vi "Periodic Tasks.vi"(8 "error in":errorcluster) -> ()   [LabVIEW 2017]
doc: "This VI runs in parallel to other tasks. It can contain as many user-defined periodic loops as you need. These can carry out PID or other sorts of timed response."
uses:
  <vilib>/Rock Robotics/WPI/DriverStation/WPI_DriverStationRobotMode2.ctl
  <vilib>/Rock Robotics/WPI/Solenoid/WPI_SolenoidValue.ctl
  <vilib>/Rock Robotics/WPI/ThirdParty/Phoenix-LabVIEW/Motor Controller/Controls/CTRE_Phoenix_MotorControl_ControlMode.ctl
  Robot Global Data.vi
  <vilib>/Rock Robotics/WPI/Solenoid/WPI_SolenoidSetEnum.vi
  <vilib>/addons/control/pid/pid.llb/PID (DBL).vi
  <vilib>/Rock Robotics/WPI/Utilities/WPI_GetSetVariantRefNum.vi
  <vilib>/Rock Robotics/WPI/ThirdParty/Phoenix-LabVIEW/Motor Controller/Get/CTRE_Phoenix_MotorController_GetOutputCurrent_Enhanced.vi
  <vilib>/addons/control/pid/NI_PID_pid.lvlib
panel:
  out "Distance":dbl
  out "Distance 2":dbl
  out "Angle":dbl
  out "Normalized Value":dbl
  out "Output Current":dbl
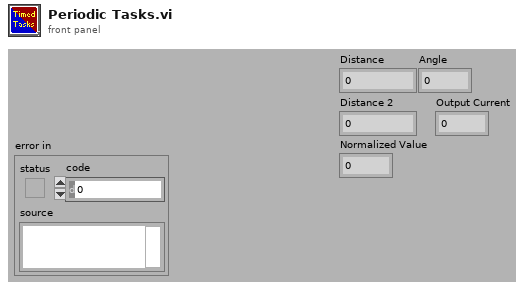
[diagram p1: front panel]
types:
  T1 = typedef "WPI_SolenoidDevRef.ctl" = cluster{"DevStatus":errorcluster, "Pneumatics Control Module":u8, "Forward Solenoid Channel":T2, "Reverse Solenoid Channel":T2}
  T2 = typedef "WPI_SolenoidChannel.ctl" = enum8{"Solenoid 0", "Solenoid 1", "Solenoid 2", "Solenoid 3", "Solenoid 4", "Solenoid 5", "Solenoid 6", "Solenoid 7", "Invalid"}
  T3 = typedef "WPI_MotorControlDeviceRef.ctl" = cluster{"DeviceStatus":errorcluster, "Type":T4, "PWM":cluster{"PWM Channel":T5, "DeadBand":T6}, "CAN":cluster{"Device Number":u8, "SetOutput VI Ref":variant, "GetOutput VI Ref":variant, "Enable VI Ref":variant, "Disable VI Ref":variant, "Data":variant}, "Invert":bool, "DIO PWM":cluster{"PWM \"Enable\" Channel":T5, "DIOChannel":T7, "PWM Rate":dbl}}
  T4 = typedef "WPI_MotorControlType.ctl" = enum16{"PWM", "CAN", "DIO PWM"}
  T5 = typedef "FPGA_DIOPWMChannel.ctl" = enum8{"PWM 0", "PWM 1", "PWM 2", "PWM 3", "PWM 4", "PWM 5", "PWM 6", "PWM 7", "PWM 8", "PWM 9", "PWM MXP 0", "PWM MXP 1", "PWM MXP 2", "PWM MXP 3", "PWM MXP 4", "PWM MXP 5", "PWM MXP 6", "PWM MXP 7", "PWM MXP 8", "PWM MXP 9", "Invalid"}
  T6 = typedef "WPI_PWMDeadband.ctl" = cluster{"Name":string, "maxPositivePwm":i32, "minPositivePwm":i32, "centerPwm":i32, "maxNegativePwm":i32, "minNegativePwm":i32, "angularRange":u16}
  T7 = typedef "FPGA_DIOChannel.ctl" = enum8{"DIO 0", "DIO 1", "DIO 2", "DIO 3", "DIO 4", "DIO 5", "DIO 6", "DIO 7", "DIO 8", "DIO 9", "DIO MXP 0", "DIO MXP 1", "DIO MXP 2", "DIO MXP 3", "DIO MXP 4", "DIO MXP 5", "DIO MXP 6", "DIO MXP 7", "DIO MXP 8", "DIO MXP 9", "DIO MXP 10", "DIO MXP 11", "DIO MXP 12", "DIO MXP 13", "DIO MXP 14", "DIO MXP 15", "SPI Port CS1", "SPI Port CS2", "SPI Port CS3", "SPI Port MISO", "SPI Port MOSI", "Invalid"}
  T8 = typedef "WPI_EncoderDevRef.ctl" = cluster{"DevStatus":errorcluster, "EncoderIndex":T9, "CounterIndex":T10, "DistancePerCount":dbl, "Decoding Type":T11}
  T9 = typedef "FPGA_EncoderIdx.ctl" = enum8{"Enc 0", "Enc 1", "Enc 2", "Enc 3", "Enc 4", "Enc 5", "Enc 6", "Enc 7", "Invalid"}
  T10 = typedef "FPGA_CounterCtrSystemIndex.ctl" = enum8{"Ctr 0", "Ctr 1", "Ctr 2", "Ctr 3", "Ctr 4", "Ctr 5", "Ctr 6", "Ctr 7", "Invalid"}
  T11 = typedef "WPI_EncoderType.ctl" = enum16{"1x", "2x", "4x"}
  T12 = typedef "WPI_JoystickDevRef.ctl" = cluster{"Device":T13}
  T13 = typedef "WPI_JoystickDeviceEnum.ctl" = enum16{"USB 0", "USB 1", "USB 2", "USB 3", "USB 4", "USB 5"}
  T14 = typedef "WPI_SolenoidValue.ctl" = enum16{"Off", "On", "Forward", "Reverse"}
  T15 = cluster{"Axes[0]":dbl, "Axes[1]":dbl, "Axes[2]":dbl, "Axes[3]":dbl, "Axes[4]":dbl, "Axes[5]":dbl, "Axes[6]":dbl, "Axes[7]":dbl, "Axes[8]":dbl}
  T16 = cluster{"X Center":i32, "X Tolerance":i32, "Y Center":i32, "Y Tolderance":i32}
  T17 = typedef "WPI_DriverStationRobotMode2.ctl" = enum16{"Autonomous Disabled", "Autonomous Enabled", "Teleop Disabled", "Teleop Enabled", "Disconnected", "Finish", "Test Disabled", "Test Enabled", "Emergency Stopped"}
  T18 = typedef "CTRE_Phoenix_MotorControl_ControlMode.ctl" = u16
  T19 = typedef "WPI_PotentiometerDevRef.ctl" = cluster{"DevStatus":errorcluster, "Analog Channel":T20, "Invert Output":bool}
  T20 = typedef "FPGA_AIChannel.ctl" = enum8{"AI 0", "AI 1", "AI 2", "AI 3", "AI MXP 0", "AI MXP 1", "AI MXP 2", "AI MXP 3", "Invalid"}
  T21 = typedef "WPI_GyroDevRef.ctl" = cluster{"DevStatus":errorcluster, "Analog Channel":T20, "Gain (VoltsPerDegree/Second)":dbl, "Gyro Type":enum16{"Analog", "XRS450"}, "Handle":i32, "SPI Bus":T22, "Device Found":bool, "Sample Rate":dbl, "Calibrate On Open":bool, "Offset":dbl}
  T22 = typedef "spi_bus.ctl" = enum16{"SPI On-Board, CS0", "SPI On-Board, CS1", "SPI On-Board, CS2", "SPI On-Board, CS3", "SPI MXP", "Invalid"}
  T23 = cluster{"proportional gain (Kc)":dbl, "integral time (Ti, min)":dbl, "derivative time (Td, min)":dbl}
  T24 = cluster{"Lower Limit":dbl, "Lower Position":dbl, "Switch":dbl, "Scale":dbl, "Upper Limit":dbl}
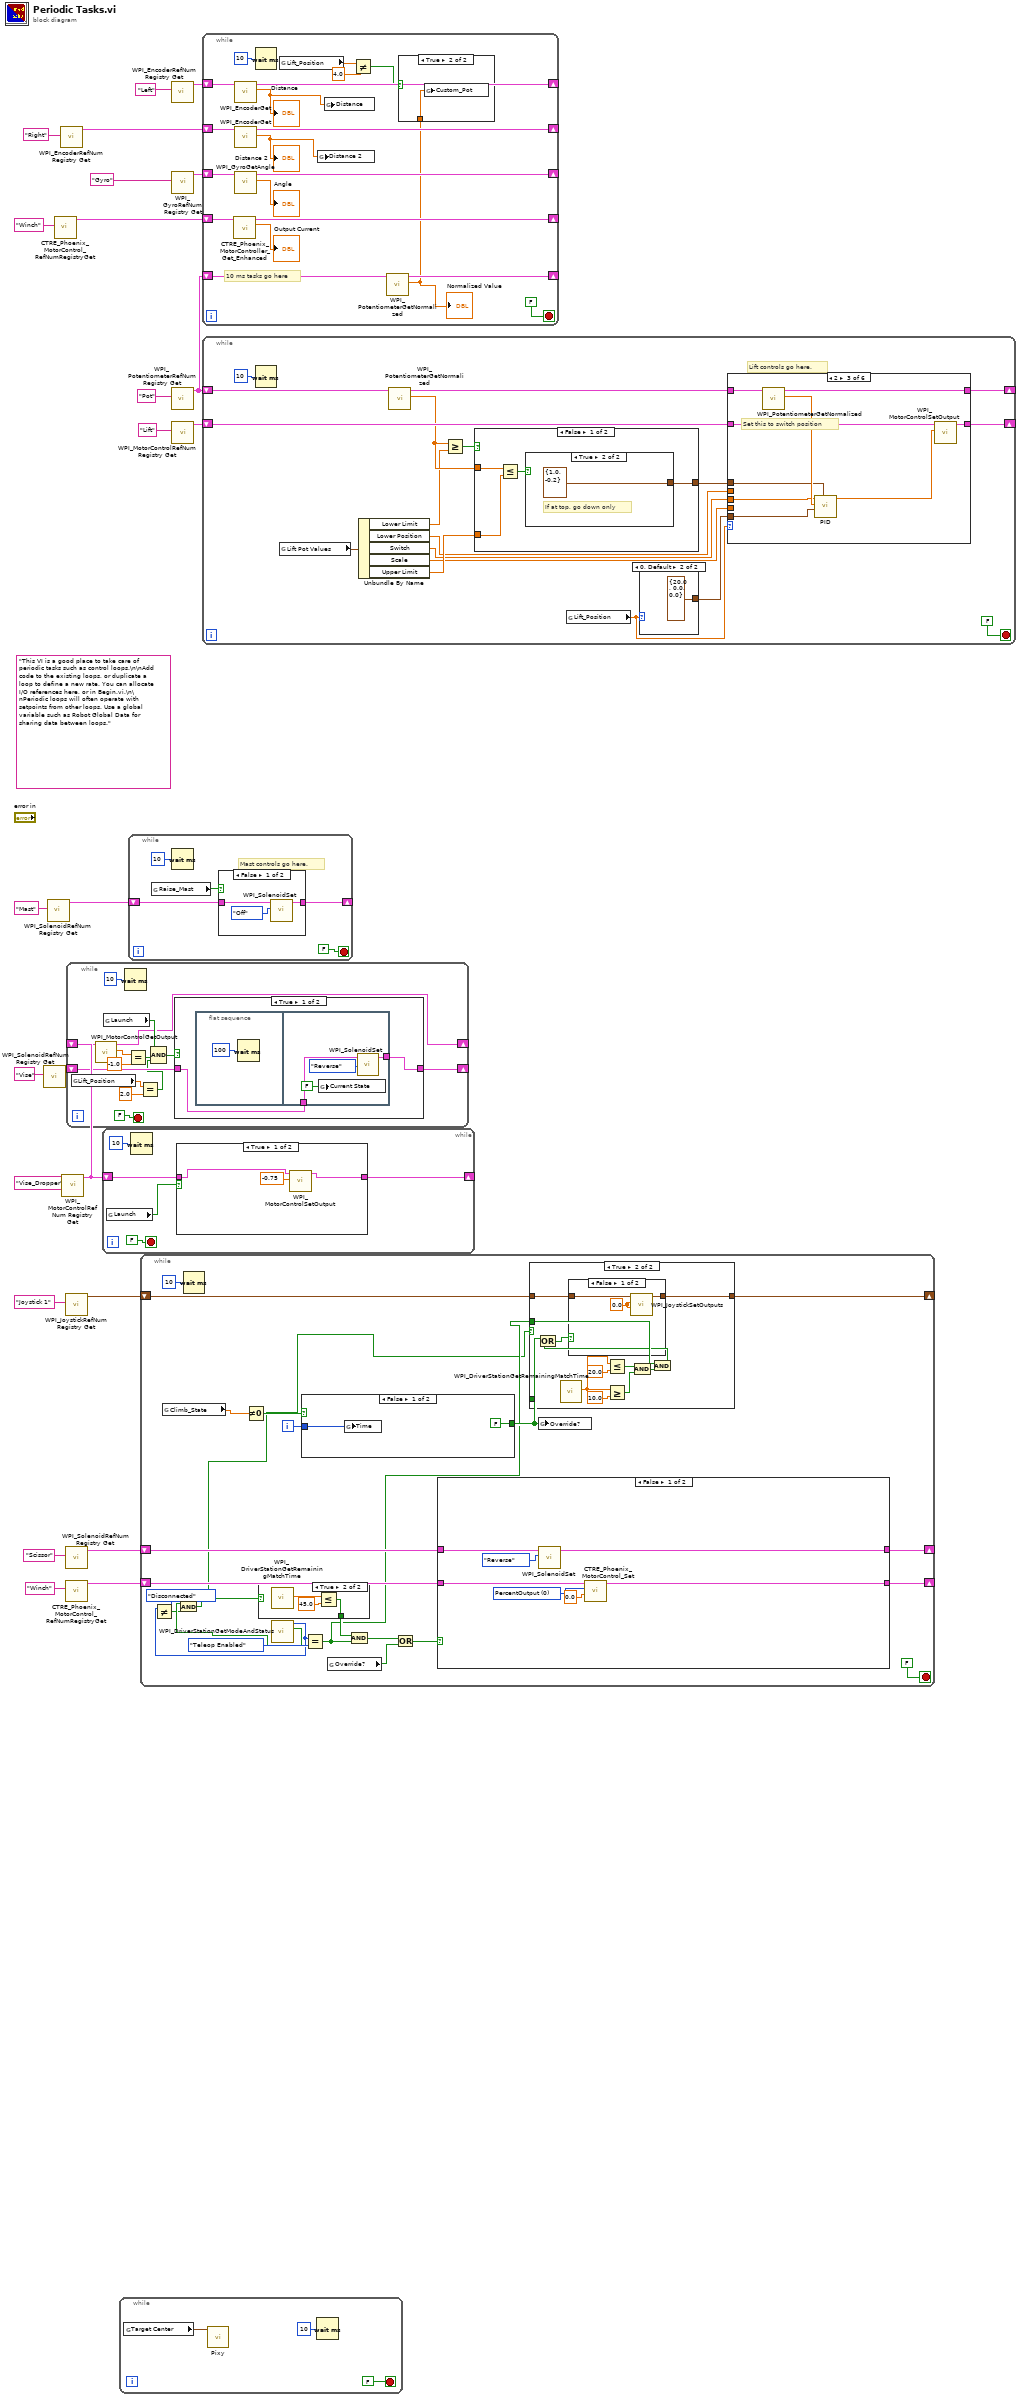
[diagram p0: block diagram]
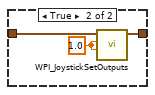
[diagram p4: hidden frame]
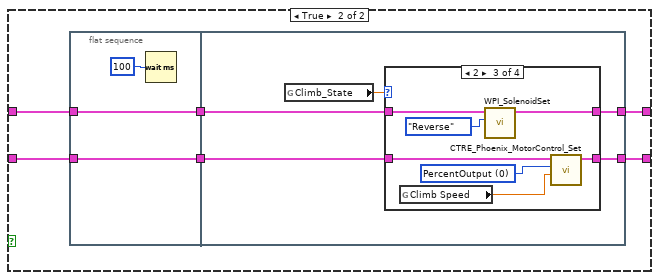
[diagram p6: hidden frame]
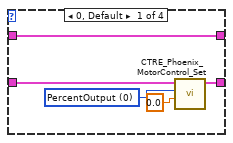
[diagram p7: hidden frame]
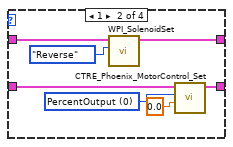
[diagram p8: hidden frame]
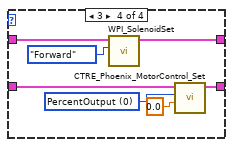
[diagram p9: hidden frame]
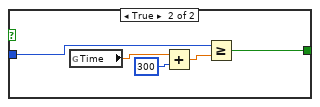
[diagram p10: hidden frame]
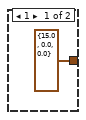
[diagram p11: hidden frame]
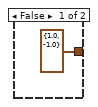
[diagram p12: hidden frame]
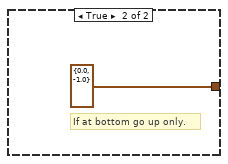
[diagram p13: hidden frame]
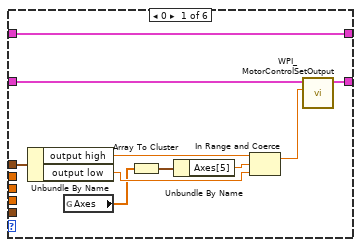
[diagram p14: hidden frame]
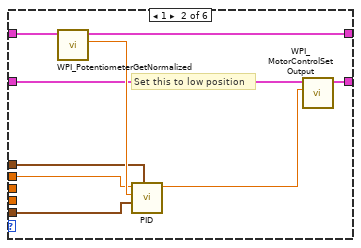
[diagram p15: hidden frame]
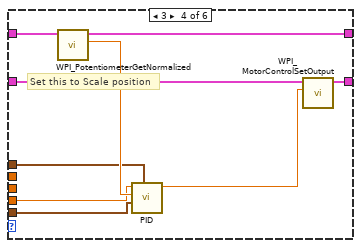
[diagram p16: hidden frame]
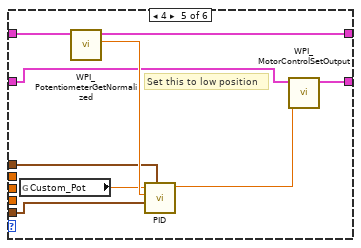
[diagram p17: hidden frame]
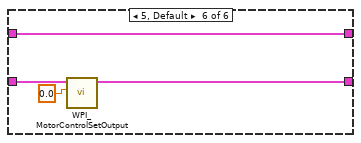
[diagram p18: hidden frame]
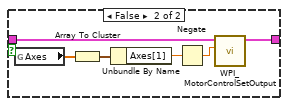
[diagram p19: hidden frame]
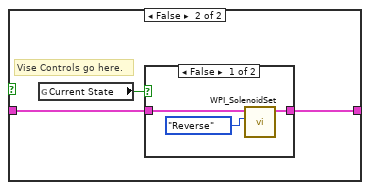
[diagram p20: hidden frame]
diagram:
  (unwired) "This VI is a good place to take care of periodic tasks such as control loops.\n\nAdd code to the existing loops, or duplicate a loop to define a new rate. You can allocate I/O references here, or in Begin.vi.\n\nPeriodic loops will often operate with setpoints from other loops. Use a global variable such as Robot Global Data for sharing data between loops."
  n1 = call <vilib>:"WPI_SolenoidRefNum Registry Get.vi"("refnum name"="Vise") -> ("SolenoidDevRef"=w21:T1)  [unwired: 9 in, 1 out]
  n2 = call <vilib>:"WPI_SolenoidRefNum Registry Get.vi"("refnum name"="Mast") -> ("SolenoidDevRef"=w23:T1)  [unwired: 9 in, 1 out]
  n3 = call <vilib>:"CTRE_Phoenix_MotorControl_RefNumRegistryGet.vi"("refnum name"="Winch") -> ("PhoenixMotorControlDevRef"=w2:T3)  [unwired: 9 in, 1 out]
  n4 = call <vilib>:"WPI_EncoderRefNum Registry Get.vi"("refnum name"="Right") -> ("EncoderDevRef"=w5:T8)  [unwired: 9 in, 1 out]
  n5 = call <vilib>:"WPI_MotorControlRefNum Registry Get.vi"("refnum name"="Vise_Dropper") -> ("MotorControlDevRef"=w1:T3)  [unwired: 9 in, 1 out]
  n6 = call <vilib>:"WPI_JoystickRefNum Registry Get.vi"("refnum name"="Joystick 1") -> ("JoystickDevRef"=w14:T12)  [unwired: 1 in, 9 out]
  n7 = call <vilib>:"WPI_SolenoidRefNum Registry Get.vi"("refnum name"="Scissor") -> ("SolenoidDevRef"=w12:T1)  [unwired: 9 in, 1 out]
  n8 = call <vilib>:"CTRE_Phoenix_MotorControl_RefNumRegistryGet.vi"("refnum name"="Winch") -> ("PhoenixMotorControlDevRef"=w10:T3)  [unwired: 9 in, 1 out]
  n9 = while {
    shift-right: [w35] -> _
    shift-left: w21 -> [w36]
    shift-right: [w31] -> _
    shift-left: w1 -> [w32]
    stop <- FALSE stop-if-true
    n10 = global read "Robot Global Data.vi" "Lift_Position"() -> (w27:dbl)
    n11 = call <vilib>:"WPI_MotorControlGetOutput.vi"("MotorControlDevRef"=w32) -> ("Output"=w30:dbl, "MotorControlDevRef"=w31:T3)  [unwired: 8 in, 1 out]
    n12 = global read "Robot Global Data.vi" "Launch"() -> (w33:bool)
    n13 = Wait (ms)(milliseconds to wait=u32 10) -> ()  [unwired: 1 out]
    n14 = Equal?(x=w30, y=-1.0) -> (x = y?=w29:bool)
    n15 = Equal?(x=w27, y=2.0) -> (x = y?=w25:bool)
    n16 = Compound Arithmetic op=AND(w33, w29, w25) -> (w34:bool)
    n17 = case shown="True" w34 {
      tunnel: w36 -> [w40 w48]
      tunnel: [w39 w47] -> w35
      frame True {
        n18 = flat-sequence {
          tunnel: w40 -> [w44]
          tunnel: [w43] -> w39
          frame #0 {
            n19 = Wait (ms)(milliseconds to wait=u32 100) -> ()  [unwired: 1 out]
          }
          frame #1 {
            n20 = global write "Robot Global Data.vi" "Current State"(FALSE ("Current State")) -> ()
            n21 = call-poly <vilib>:"WPI_SolenoidSet.vi"("Value"=WPI_SolenoidValue."Reverse", "SolenoidDevRef"=w44) -> ("SolenoidDevRef"=w43:T1)  [unwired: 8 in, 1 out]
          }
        }
      }
      frame False {
        # "Vise Controls go here."
        n22 = global read "Robot Global Data.vi" "Current State"() -> (w46:bool)
        n23 = case shown="False" w46 {
          tunnel: [w49 w54] -> w47
          tunnel: w48 -> [w50 w52]
          frame False {
            n24 = call-poly <vilib>:"WPI_SolenoidSet.vi"("Value"=WPI_SolenoidValue."Reverse", "SolenoidDevRef"=w50) -> ("SolenoidDevRef"=w49:T1)  [unwired: 8 in, 1 out]
          }
          frame True {
            n25 = call-poly <vilib>:"WPI_SolenoidSet.vi"("Value"=WPI_SolenoidValue."Forward", "SolenoidDevRef"=w52) -> ("SolenoidDevRef"=w54:T1)  [unwired: 8 in, 1 out]
          }
        }
      }
    }
  }
  n26 = while {
    shift-right: [w56] -> _
    shift-left: w1 -> [w57]
    stop <- FALSE stop-if-true
    n27 = global read "Robot Global Data.vi" "Launch"() -> (w55:bool)
    n28 = Wait (ms)(milliseconds to wait=u32 10) -> ()  [unwired: 1 out]
    n29 = case shown="True" w55 {
      tunnel: w57 -> [w61 w65]
      tunnel: [w60 w64] -> w56
      frame True {
        n30 = call <vilib>:"WPI_MotorControlSetOutput.vi"("Output"=-0.75, "MotorControlDevRef"=w61) -> ("MotorControlDevRef"=w60:T3)  [unwired: 7 in, 2 out]
      }
      frame False {
        n31 = global read "Robot Global Data.vi" "Axes"() -> (w63:dbl[])
        n32 = Array To Cluster(array=w63) -> (cluster=w68:T15)
        n33 = Unbundle By Name(w68) -> ("Axes[1]"=w67:dbl)
        n34 = Negate(x=w67) -> (-x=w66:dbl)
        n35 = call <vilib>:"WPI_MotorControlSetOutput.vi"("Output"=w66, "MotorControlDevRef"=w65) -> ("MotorControlDevRef"=w64:T3)  [unwired: 7 in, 2 out]
      }
    }
  }
  n36 = while {
    stop <- FALSE stop-if-true
    n37 = global read "Robot Global Data.vi" "Target Center"() -> (w69:T16)
    n38 = call "Pixy.vi"("Target Center"=w69) -> ()  [unwired: 11 in]
    n39 = Wait (ms)(milliseconds to wait=u32 10) -> ()  [unwired: 1 out]
  }
  n40 = while {
    shift-right: [w73] -> _
    shift-left: w23 -> [w74]
    stop <- FALSE stop-if-true
    # "Mast controls go here."
    n41 = global read "Robot Global Data.vi" "Raise_Mast"() -> (w72:bool)
    n42 = Wait (ms)(milliseconds to wait=u32 10) -> ()  [unwired: 1 out]
    n43 = case shown="False" w72 {
      tunnel: w74 -> [w78 w82]
      tunnel: [w77 w81] -> w73
      frame False {
        n44 = call-poly <vilib>:"WPI_SolenoidSet.vi"("Value"=WPI_SolenoidValue."Off", "SolenoidDevRef"=w78) -> ("SolenoidDevRef"=w77:T1)  [unwired: 8 in, 1 out]
      }
      frame True {
        n45 = call-poly <vilib>:"WPI_SolenoidSet.vi"("Value"=WPI_SolenoidValue."On", "SolenoidDevRef"=w82) -> ("SolenoidDevRef"=w81:T1)  [unwired: 8 in, 1 out]
      }
    }
  }
  n46 = while {
    shift-right: [w96] -> _
    shift-left: w14 -> [w97]
    shift-right: [w94] -> _
    shift-left: w12 -> [w95]
    shift-right: [w92] -> _
    shift-left: w10 -> [w93]
    i -> [w98]
    stop <- FALSE stop-if-true
    n47 = global read "Robot Global Data.vi" "Climb_State"() -> (w83:dbl)
    n48 = Wait (ms)(milliseconds to wait=u32 10) -> ()  [unwired: 1 out]
    n49 = Not Equal To 0?(x=w83) -> (x != 0?=w99:bool)
    n50 = call <vilib>:"WPI_DriverStationGetModeAndStatus.vi"() -> ("FMS Attached"=w87:bool, "Robot Mode"=w85:T17)  [unwired: 10 in]
    n51 = Not Equal?(x=w85, y=WPI_DriverStationRobotMode2."Disconnected") -> (x != y?=w86:bool)
    n52 = And(x=w87, y=w86) -> (x .and. y?=w88:bool)
    n53 = case shown="True" w88 {
      selector: w88 -> [w125 _]
      tunnel: [w125 w127] -> w103
      frame False {
      }
      frame True {
        n54 = call <vilib>:"WPI_DriverStationGetRemainingMatchTime.vi"() -> ("Match Time(s)"=w126:sgl)  [unwired: 10 in, 1 out]
        n55 = Less Or Equal?(x=w126, y=sgl 45.0) -> (x <= y?=w127:bool)
      }
    }
    n56 = case shown="False" w99 {
      tunnel: w98 -> [w176 w179]
      tunnel: [FALSE w181] -> w91
      frame False {
        n57 = global write "Robot Global Data.vi" "Time"(w176) -> ()
      }
      frame True {
        n58 = global read "Robot Global Data.vi" "Time"() -> (w178:dbl)
        n59 = Add(x=w178, y=300) -> (x+y=w180:dbl)
        n60 = Greater Or Equal?(x=w179, y=w180) -> (x >= y?=w181:bool)
      }
    }
    n61 = Equal?(x=w85, y=WPI_DriverStationRobotMode2."Teleop Enabled") -> (x = y?=w89:bool)
    n62 = global read "Robot Global Data.vi" "Override?"() -> (w90:bool)
    n63 = And(x=w103, y=w89) -> (x .and. y?=w101:bool)
    n64 = Or(x=w101, y=w90) -> (x .or. y?=w100:bool)
    n65 = case shown="False" w100 {
      tunnel: w95 -> [w135 w141]
      tunnel: [w134 w140] -> w94
      tunnel: w93 -> [w130 w139]
      tunnel: [w129 w138] -> w92
      frame False {
        w132 = T18 0 items=["PercentOutput"=0, "Position"=1, "Velocity"=2, "Current"=3, "Follower"=5, "MotionProfile"=6, "MotionMagic"=7, "MotionMagicArc"=8, "MotionProfileArc"=10, "Disabled"=15] ("Control Mode")
        n66 = call-poly <vilib>:"WPI_SolenoidSet.vi"("Value"=WPI_SolenoidValue."Reverse", "SolenoidDevRef"=w135) -> ("SolenoidDevRef"=w134:T1)  [unwired: 8 in, 1 out]
        n67 = call <vilib>:"CTRE_Phoenix_MotorControl_Set.vi"("Output"=0.0, "Control Mode"=w132, "PhoenixMotorControlDevRef"=w130) -> ("PhoenixMotorControlDevRef"=w129:T3)  [unwired: 7 in, 1 out]
      }
      frame True {
        n68 = flat-sequence {
          tunnel: w139 -> [w143]
          tunnel: w141 -> [w144]
          tunnel: [w144] -> w137
          tunnel: [w143] -> w136
          tunnel: [w148] -> w140
          tunnel: [w146] -> w138
          tunnel: w137 -> [w149]
          tunnel: w136 -> [w147]
          frame #0 {
            n69 = Wait (ms)(milliseconds to wait=u32 100) -> ()  [unwired: 1 out]
          }
          frame #1 {
            n70 = global read "Robot Global Data.vi" "Climb_State"() -> (w145:dbl)
            n71 = case shown="2" w145 {
              tunnel: w149 -> [w154 w161 w168 w175]
              tunnel: [w154 w159 w167 w174] -> w148
              tunnel: w147 -> [w151 w156 w165 w170]
              tunnel: [w150 w155 w164 w169] -> w146
              frame 0, Default {
                w153 = T18 0 items=["PercentOutput"=0, "Position"=1, "Velocity"=2, "Current"=3, "Follower"=5, "MotionProfile"=6, "MotionMagic"=7, "MotionMagicArc"=8, "MotionProfileArc"=10, "Disabled"=15] ("Control Mode")
                n72 = call <vilib>:"CTRE_Phoenix_MotorControl_Set.vi"("Output"=0.0, "Control Mode"=w153, "PhoenixMotorControlDevRef"=w151) -> ("PhoenixMotorControlDevRef"=w150:T3)  [unwired: 7 in, 1 out]
              }
              frame 1 {
                w158 = T18 0 items=["PercentOutput"=0, "Position"=1, "Velocity"=2, "Current"=3, "Follower"=5, "MotionProfile"=6, "MotionMagic"=7, "MotionMagicArc"=8, "MotionProfileArc"=10, "Disabled"=15] ("Control Mode")
                n73 = call-poly <vilib>:"WPI_SolenoidSet.vi"("Value"=WPI_SolenoidValue."Reverse", "SolenoidDevRef"=w161) -> ("SolenoidDevRef"=w159:T1)  [unwired: 8 in, 1 out]
                n74 = call <vilib>:"CTRE_Phoenix_MotorControl_Set.vi"("Output"=0.0, "Control Mode"=w158, "PhoenixMotorControlDevRef"=w156) -> ("PhoenixMotorControlDevRef"=w155:T3)  [unwired: 7 in, 1 out]
              }
              frame 2 {
                w163 = T18 0 items=["PercentOutput"=0, "Position"=1, "Velocity"=2, "Current"=3, "Follower"=5, "MotionProfile"=6, "MotionMagic"=7, "MotionMagicArc"=8, "MotionProfileArc"=10, "Disabled"=15] ("Control Mode")
                n75 = global read "Robot Global Data.vi" "Climb Speed"() -> (w162:dbl)
                n76 = call-poly <vilib>:"WPI_SolenoidSet.vi"("Value"=WPI_SolenoidValue."Reverse", "SolenoidDevRef"=w168) -> ("SolenoidDevRef"=w167:T1)  [unwired: 8 in, 1 out]
                n77 = call <vilib>:"CTRE_Phoenix_MotorControl_Set.vi"("Output"=w162, "Control Mode"=w163, "PhoenixMotorControlDevRef"=w165) -> ("PhoenixMotorControlDevRef"=w164:T3)  [unwired: 7 in, 1 out]
              }
              frame 3 {
                w172 = T18 0 items=["PercentOutput"=0, "Position"=1, "Velocity"=2, "Current"=3, "Follower"=5, "MotionProfile"=6, "MotionMagic"=7, "MotionMagicArc"=8, "MotionProfileArc"=10, "Disabled"=15] ("Control Mode")
                n78 = call-poly <vilib>:"WPI_SolenoidSet.vi"("Value"=WPI_SolenoidValue."Forward", "SolenoidDevRef"=w175) -> ("SolenoidDevRef"=w174:T1)  [unwired: 8 in, 1 out]
                n79 = call <vilib>:"CTRE_Phoenix_MotorControl_Set.vi"("Output"=0.0, "Control Mode"=w172, "PhoenixMotorControlDevRef"=w170) -> ("PhoenixMotorControlDevRef"=w169:T3)  [unwired: 7 in, 1 out]
              }
            }
          }
        }
      }
    }
    n80 = case shown="True" w88 {
      tunnel: w89 -> [_ w118]
      tunnel: w97 -> [w106 w115]
      tunnel: [w106 w114] -> w96
      tunnel: w91 -> [_ w113]
      frame False {
      }
      frame True {
        n81 = call <vilib>:"WPI_DriverStationGetRemainingMatchTime.vi"() -> ("Match Time(s)"=w107:sgl)  [unwired: 10 in, 1 out]
        n82 = Less Or Equal?(x=w107, y=sgl 20.0) -> (x <= y?=w111:bool)
        n83 = Greater Or Equal?(x=w107, y=sgl 10.0) -> (x >= y?=w110:bool)
        n84 = And(x=w111, y=w110) -> (x .and. y?=w108:bool)
        n85 = And(x=w118, y=w108) -> (x .and. y?=w117:bool)
        n86 = Or(x=w113, y=w117) -> (x .or. y?=w116:bool)
        n87 = case shown="False" w116 {
          tunnel: w115 -> [w120 w124]
          tunnel: [w119 w123] -> w114
          frame False {
            w121 = sgl 0.0 ("Left Rumble")
            n88 = call <vilib>:"WPI_JoystickSetOutputs.vi"("Right Rumble"=w121, "Left Rumble"=w121, "JoystickDevRef"=w120) -> ("JoystickDevRef"=w119:T12)  [unwired: 7 in, 1 out]
          }
          frame True {
            w122 = sgl 1.0 ("Left Rumble")
            n89 = call <vilib>:"WPI_JoystickSetOutputs.vi"("Right Rumble"=w122, "Left Rumble"=w122, "JoystickDevRef"=w124) -> ("JoystickDevRef"=w123:T12)  [unwired: 7 in, 1 out]
          }
        }
      }
    }
    n90 = global write "Robot Global Data.vi" "Override?"(w91) -> ()
  }
  n91 = call <vilib>:"WPI_EncoderRefNum Registry Get.vi"("refnum name"="Left") -> ("EncoderDevRef"=w4:T8)  [unwired: 9 in, 1 out]
  n92 = call <vilib>:"WPI_PotentiometerRefNum Registry Get.vi"("refnum name"="Pot") -> ("PotDevRef"=w16:T19)  [unwired: 9 in, 1 out]
  n93 = call <vilib>:"WPI_GyroRefNum Registry Get.vi"("refnum name"="Gyro") -> ("GyroDevRef"=w6:T21)  [unwired: 9 in, 1 out]
  n94 = call <vilib>:"WPI_MotorControlRefNum Registry Get.vi"("refnum name"="Lift") -> ("MotorControlDevRef"=w18:T3)  [unwired: 9 in, 1 out]
  n95 = while {
    shift-right: [w197] -> _
    shift-left: w6 -> [w200]
    shift-right: [w196] -> _
    shift-left: w5 -> [w199]
    shift-right: [w195] -> _
    shift-left: w4 -> [w198]
    shift-right: [w192] -> _
    shift-left: w16 -> [w193]
    shift-right: [w190] -> _
    shift-left: w2 -> [w191]
    stop <- FALSE stop-if-true
    # "10 ms tasks go here"
    n96 = call-poly <vilib>:"CTRE_Phoenix_MotorController_Get_Enhanced.vi"("PhoenixMotorControlDevRef"=w191) -> ("PhoenixMotorControlDevRef"=w190:T3, "Output Current"=→"Output Current":dbl)  [unwired: 12 in, 1 out]
    n97 = call <vilib>:"WPI_EncoderGet.vi"("EncoderDevRef"=w198) -> ("Distance"=w184:dbl, "EncoderDevRef"=w195:T8)  [unwired: 5 in, 4 out]
    "Distance" <- w184
    n98 = call <vilib>:"WPI_EncoderGet.vi"("EncoderDevRef"=w199) -> ("Distance"=w183:dbl, "EncoderDevRef"=w196:T8)  [unwired: 5 in, 4 out]
    "Distance 2" <- w183
    n99 = call <vilib>:"WPI_GyroGetAngle.vi"("GyroDevRef"=w200) -> ("Angle"=→"Angle":dbl, "GyroDevRef"=w197:T21)  [unwired: 6 in, 3 out]
    n100 = Wait (ms)(milliseconds to wait=u32 10) -> ()  [unwired: 1 out]
    n101 = global read "Robot Global Data.vi" "Lift_Position"() -> (w188:dbl)
    n102 = global write "Robot Global Data.vi" "Distance 2"(w183) -> ()
    n103 = global write "Robot Global Data.vi" "Distance"(w184) -> ()
    n104 = Not Equal?(x=w188, y=4.0) -> (x != y?=w186:bool)
    n105 = call <vilib>:"WPI_PotentiometerGetNormalized.vi"("PotDevRef"=w193) -> ("Normalized Value"=w185:dbl, "PotDevRef"=w192:T19)  [unwired: 8 in, 1 out]
    "Normalized Value" <- w185
    n106 = case shown="True" w186 {
      tunnel: w185 -> [_ w203]
      frame False {
      }
      frame True {
        n107 = global write "Robot Global Data.vi" "Custom_Pot"(w203) -> ()
      }
    }
  }
  n108 = while {
    shift-right: [w218] -> _
    shift-left: w18 -> [w219]
    shift-right: [w217] -> _
    shift-left: w16 -> [w214]
    stop <- FALSE stop-if-true
    # "Lift controls go here."
    n109 = Wait (ms)(milliseconds to wait=u32 10) -> ()  [unwired: 1 out]
    n110 = global read "Robot Global Data.vi" "Lift Pot Values"() -> (w209:T24)
    n111 = Unbundle By Name(w209) -> ("Lower Limit"=w208:dbl, "Lower Position"=w206:dbl, "Switch"=w205:dbl, "Scale"=w204:dbl, "Upper Limit"=w207:dbl)
    n112 = call <vilib>:"WPI_PotentiometerGetNormalized.vi"("PotDevRef"=w214) -> ("Normalized Value"=w212:dbl, "PotDevRef"=w213:T19)  [unwired: 8 in, 1 out]
    n113 = Greater Or Equal?(x=w212, y=w208) -> (x >= y?=w215:bool)
    n114 = case shown="False" w215 {
      tunnel: [w227 cluster{"output high":dbl, "output low":dbl} {"output high"=0.0, "output low"=-1.0} ("output range")] -> w216
      tunnel: w212 -> [w225 _]
      tunnel: w207 -> [w224 _]
      frame False {
        n115 = Less Or Equal?(x=w225, y=w224) -> (x <= y?=w226:bool)
        n116 = case shown="True" w226 {
          tunnel: [cluster{"output high":dbl, "output low":dbl} {"output high"=1.0, "output low"=-1.0} ("output range") cluster{"output high":dbl, "output low":dbl} {"output high"=1.0, "output low"=-0.2} ("output range")] -> w227
          frame False {
          }
          frame True {
            # "If at top, go down only"
          }
        }
      }
      frame True {
        # "If at bottom go up only."
      }
    }
    n117 = global read "Robot Global Data.vi" "Lift_Position"() -> (w210:dbl)
    n118 = case shown="0, Default" w210 {
      tunnel: [T23 {"proportional gain (Kc)"=15.0, "integral time (Ti, min)"=0.0, "derivative time (Td, min)"=0.0} ("PID gains") T23 {"proportional gain (Kc)"=20.0, "integral time (Ti, min)"=0.0, "derivative time (Td, min)"=0.0} ("PID gains")] -> w211
      frame 1 {
      }
      frame 0, Default {
      }
    }
    n119 = case shown="2" w210 {
      tunnel: w219 -> [w238 w246 w255 w264 w272 w278]
      tunnel: [w237 w245 w254 w263 w271 w277] -> w218
      tunnel: w213 -> [w239 w249 w257 w266 w274 w280]
      tunnel: [w239 w247 w256 w265 w273 w280] -> w217
      tunnel: w216 -> [w235 w243 w252 w259 w269 _]
      tunnel: w211 -> [_ w242 w251 w261 w270 _]
      tunnel: w206 -> [_ w241 _ _ _ _]
      tunnel: w205 -> [_ _ w250 _ _ _]
      tunnel: w204 -> [_ _ _ w260 _ _]
      frame 0 {
        n120 = Unbundle By Name(w235) -> ("output high"=w234:dbl, "output low"=w233:dbl)
        n121 = global read "Robot Global Data.vi" "Axes"() -> (w231:dbl[])
        n122 = Array To Cluster(array=w231) -> (cluster=w240:T15)
        n123 = Unbundle By Name(w240) -> ("Axes[5]"=w236:dbl)
        n124 = In Range and Coerce(upper limit=w234, x=w236, lower limit=w233) -> (coerced(x)=w232:dbl)  [unwired: 1 out]
        n125 = call <vilib>:"WPI_MotorControlSetOutput.vi"("Output"=w232, "MotorControlDevRef"=w238) -> ("MotorControlDevRef"=w237:T3)  [unwired: 7 in, 2 out]
      }
      frame 1 {
        # "Set this to low position"
        n126 = call <vilib>:"WPI_PotentiometerGetNormalized.vi"("PotDevRef"=w249) -> ("Normalized Value"=w248:dbl, "PotDevRef"=w247:T19)  [unwired: 8 in, 1 out]
        n127 = call-poly <vilib>:"PID.vi"("output range"=w243, "PID gains"=w242, "process variable"=w248, "setpoint"=w241) -> ("output"=w244:dbl)  [unwired: 6 in, 1 out]
        n128 = call <vilib>:"WPI_MotorControlSetOutput.vi"("Output"=w244, "MotorControlDevRef"=w246) -> ("MotorControlDevRef"=w245:T3)  [unwired: 7 in, 2 out]
      }
      frame 2 {
        # "Set this to switch position"
        n129 = call <vilib>:"WPI_PotentiometerGetNormalized.vi"("PotDevRef"=w257) -> ("Normalized Value"=w258:dbl, "PotDevRef"=w256:T19)  [unwired: 8 in, 1 out]
        n130 = call-poly <vilib>:"PID.vi"("output range"=w252, "PID gains"=w251, "process variable"=w258, "setpoint"=w250) -> ("output"=w253:dbl)  [unwired: 6 in, 1 out]
        n131 = call <vilib>:"WPI_MotorControlSetOutput.vi"("Output"=w253, "MotorControlDevRef"=w255) -> ("MotorControlDevRef"=w254:T3)  [unwired: 7 in, 2 out]
      }
      frame 3 {
        # "Set this to Scale position"
        n132 = call <vilib>:"WPI_PotentiometerGetNormalized.vi"("PotDevRef"=w266) -> ("Normalized Value"=w267:dbl, "PotDevRef"=w265:T19)  [unwired: 8 in, 1 out]
        n133 = call-poly <vilib>:"PID.vi"("output range"=w259, "PID gains"=w261, "process variable"=w267, "setpoint"=w260) -> ("output"=w262:dbl)  [unwired: 6 in, 1 out]
        n134 = call <vilib>:"WPI_MotorControlSetOutput.vi"("Output"=w262, "MotorControlDevRef"=w264) -> ("MotorControlDevRef"=w263:T3)  [unwired: 7 in, 2 out]
      }
      frame 4 {
        # "Set this to low position"
        n135 = global read "Robot Global Data.vi" "Custom_Pot"() -> (w268:dbl)
        n136 = call <vilib>:"WPI_PotentiometerGetNormalized.vi"("PotDevRef"=w274) -> ("Normalized Value"=w276:dbl, "PotDevRef"=w273:T19)  [unwired: 8 in, 1 out]
        n137 = call-poly <vilib>:"PID.vi"("output range"=w269, "PID gains"=w270, "process variable"=w276, "setpoint"=w268) -> ("output"=w275:dbl)  [unwired: 6 in, 1 out]
        n138 = call <vilib>:"WPI_MotorControlSetOutput.vi"("Output"=w275, "MotorControlDevRef"=w272) -> ("MotorControlDevRef"=w271:T3)  [unwired: 7 in, 2 out]
      }
      frame 5, Default {
        n139 = call <vilib>:"WPI_MotorControlSetOutput.vi"("Output"=0.0, "MotorControlDevRef"=w278) -> ("MotorControlDevRef"=w277:T3)  [unwired: 7 in, 2 out]
      }
    }
  }
